vi "FlatToRichcif_manager_LauncherDestroy.vi"(5 "OutputClusterType":T1, 11 "InputCluster":T2) -> (3 "OutputCluster":T1)   [LabVIEW 2021, in "CIF_Manager_server.lvlib"]
uses:
  CIF_Manager_server.lvlib
  cif_manager_LauncherDestroy_Flat.ctl
  cif_manager_LauncherDestroy.ctl
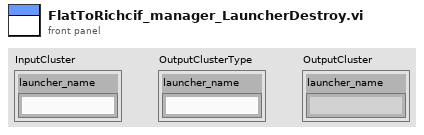
[diagram p1: front panel]
types:
  T1 = typedef "CIF_Manager_server.lvlib/cif_manager_LauncherDestroy.ctl" = cluster{"launcher_name":string}
  T2 = typedef "CIF_Manager_server.lvlib/cif_manager_LauncherDestroy_Flat.ctl" = cluster{"launcher_name":string}
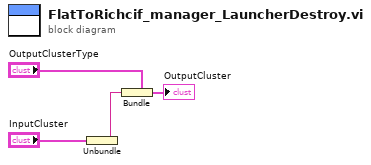
[diagram p0: block diagram]
diagram:
  n1 = Unbundle "Unbundle"("InputCluster") -> ("launcher_name"=w1:string)
  n2 = Bundle "Bundle"(cluster="OutputClusterType", "launcher_name"=w1) -> (→"OutputCluster":T1)
